vi "VIP_Pre-Install Custom Action.vi"(10 "Variant":variant) -> (0 "error out":errorcluster)   [LabVIEW 2021]
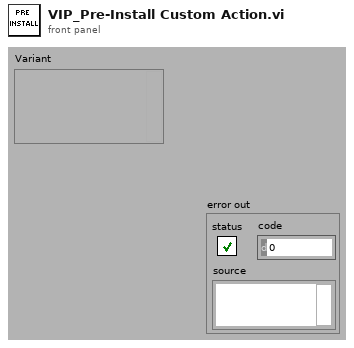
[diagram p1: front panel]
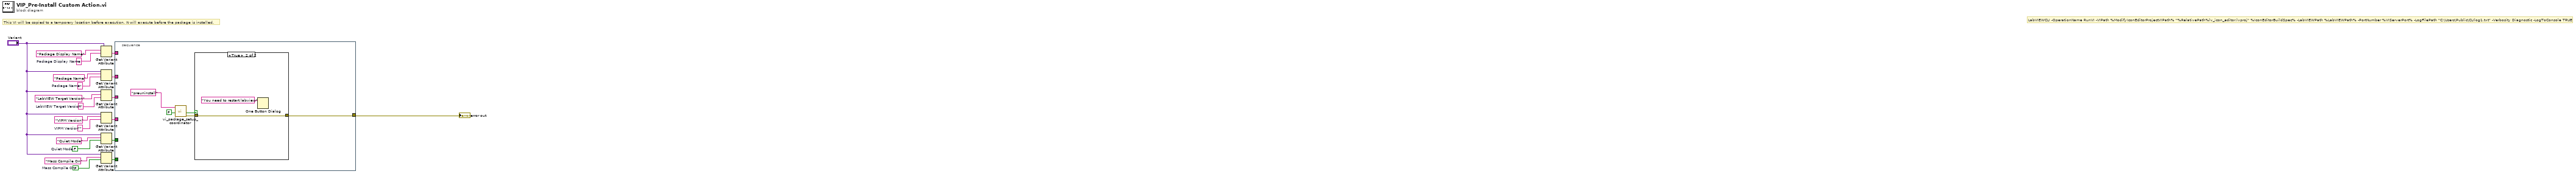
[diagram p0: block diagram]
diagram:
  w2 = FALSE  # Mass Compile On
  w4 = ""  # Package Display Name
  w11 = FALSE  # Quiet Mode
  w14 = ""  # VIPM Version
  w16 = ""  # LabVIEW Target Version
  w18 = ""  # Package Name
  # "LabVIEWCLI -OperationName RunVI -VIPath %ModifyIconEditorProjectVIPath% \"%RelativePath%lv_icon_editor.lvproj\" %IconEditorBuildSpec% -LabVIEWPath %LabVIEWPath% -PortNumber %VIServerPort% -LogFilePath \"C:\\Users\\Public\\CLIlog1.txt\" -Verbosity Diagnostic -LogToConsole TRUE"
  # "This VI will be copied to a temporary location before execution. It will execute before the package is installed."
  n1 = Get Variant Attribute(Variant="Variant", name="Package Display Name", default value (empty Variant)=w4) -> (value=w10:string)  [unwired: 1 in, 3 out]
  n2 = Get Variant Attribute(Variant="Variant", name="Package Name", default value (empty Variant)=w18) -> (value=w9:string)  [unwired: 1 in, 3 out]
  n3 = Get Variant Attribute(Variant="Variant", name="LabVIEW Target Version", default value (empty Variant)=w16) -> (value=w8:string)  [unwired: 1 in, 3 out]
  n4 = Get Variant Attribute(Variant="Variant", name="VIPM Version", default value (empty Variant)=w14) -> (value=w7:string)  [unwired: 1 in, 3 out]
  n5 = Get Variant Attribute(Variant="Variant", name="Quiet Mode", default value (empty Variant)=w11) -> (value=w6:bool)  [unwired: 1 in, 3 out]
  n6 = Get Variant Attribute(Variant="Variant", name="Mass Compile On", default value (empty Variant)=w2) -> (value=w5:bool)  [unwired: 1 in, 3 out]
  n7 = stacked-sequence {
    tunnel: w10 -> [_]
    tunnel: w9 -> [_]
    tunnel: w8 -> [_]
    tunnel: w7 -> [_]
    tunnel: w6 -> [_]
    tunnel: w5 -> [_]
    tunnel: [w21] -> w1
    frame #0 {
      n8 = call "vi_package_setup_coordinator.vi"("Set"=FALSE, "name in"="preuninstall") -> ("error out"=w22:errorcluster, "Found"=w23:bool)  [unwired: 6 in, 2 out]
      n9 = case shown="True" w23 {
        tunnel: w22 -> [w26 w27]
        tunnel: [w26 w27] -> w21
        frame False {
        }
        frame True {
          n10 = One Button Dialog(message="You need to restart labview") -> ()  [unwired: 1 in, 1 out]
        }
      }
    }
  }
  "error out" <- w1
